vi "BDF-Read Record For Playback.vi"(0 "Header":T1, 5 "refnum in":refnum<file>, 9 "TCP samples":i32, 11 "error in (no error)":errorcluster) -> (6 "refnum out":refnum<file>, 8 "Array":u8[][](array[numeric]), 15 "error out":errorcluster)   [LabVIEW 2020]
uses:
  BDF-Header.ctl
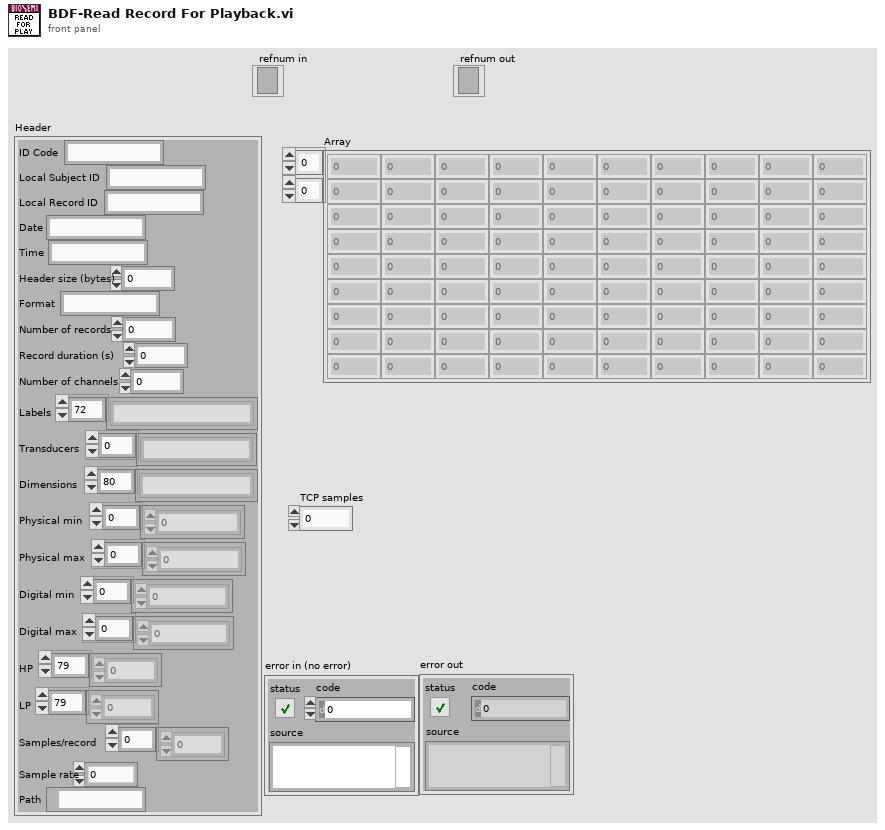
[diagram p1: front panel]
types:
  T1 = typedef "BDF-Header.ctl" = cluster{"ID Code":string, "Local Subject ID":string, "Local Record ID":string, "Date":string, "Time":string, "Header size (bytes)":i32, "Format":string, "Number of records":i32, "Record duration (s)":dbl, "Number of channels":i32, "Labels":string[], "Transducers":string[], "Dimensions":string[], "Physical min":dbl[], "Physical max":dbl[], "Digital min":i32[], "Digital max":i32[], "HP":dbl[], "LP":dbl[], "Samples/record":i32[], "Sample rate":dbl, "Path":path}
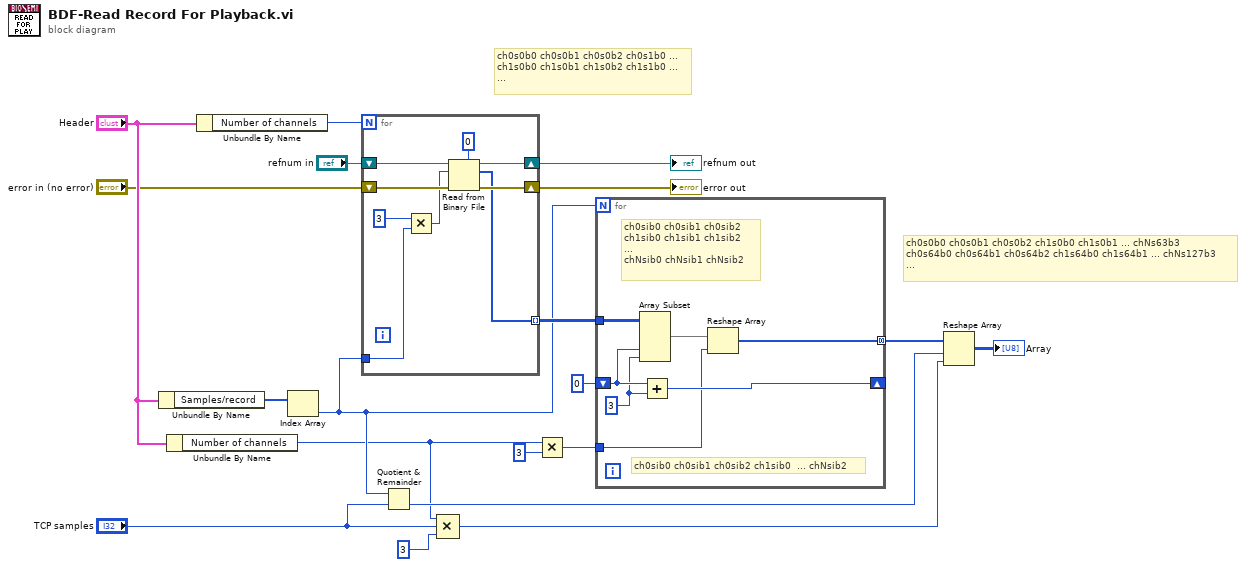
[diagram p0: block diagram]
diagram:
  # "ch0s0b0 ch0s0b1 ch0s0b2 ch1s0b0 ch1s0b1 ... chNs63b3\nch0s64b0 ch0s64b1 ch0s64b2 ch1s64b0 ch1s64b1 ... chNs127b3\n..."
  # "ch0s0b0 ch0s0b1 ch0s0b2 ch0s1b0 ...\nch1s0b0 ch1s0b1 ch1s0b2 ch1s1b0 ...\n..."
  n1 = Unbundle By Name("Header") -> ("Samples/record"=w17:i32[])
  n2 = Unbundle By Name("Header") -> ("Number of channels"=w5:i32)
  n3 = Unbundle By Name("Header") -> ("Number of channels"=w19:i32)
  n4 = Index Array(array=w17) -> (element=w6:i32)  [unwired: 1 in]
  n5 = for {
    N: w19 -> [_]
    tunnel: w6 -> [w20]
    shift-right: [w23] -> w3
    shift-left: "refnum in" -> [w28]
    shift-right: [w26] -> w1
    shift-left: "error in (no error)" -> [w27]
    tunnel: [w21] -> w8 mode=indexing
    n6 = Multiply(x=3, y=w20) -> (x*y=w24:i32)
    n7 = Read from Binary File(5:u8 0 ("Numeric"), 8:w27, 10:w24, 11:w28) -> (0:w26:errorcluster, 2:w21:u8[], 3:w23:refnum<file>)  [unwired: 2 in, 1 out]
  }
  "error out" <- w1
  "refnum out" <- w3
  n8 = Quotient & Remainder(x=w6, y="TCP samples") -> (floor(x/y)=w10:i32)  [unwired: 1 out]
  n9 = Compound Arithmetic op=MULTIPLY(w5, "TCP samples", 3 ("y")) -> (w12:i32)
  n10 = Multiply(x=w5, y=3) -> (x*y=w14:i32)
  n11 = for {
    N: w6 -> [_]
    tunnel: w8 -> [w35]
    shift-right: [w32] -> _
    shift-left: 0 -> [w34]
    tunnel: [w30] -> w7 mode=concatenating
    tunnel: w14 -> [w29]
    w33 = 3 ("length")
    # "ch0sib0 ch0sib1 ch0sib2 ch1sib0  ... chNsib2"
    # "ch0sib0 ch0sib1 ch0sib2\nch1sib0 ch1sib1 ch1sib2\n...\nchNsib0 chNsib1 chNsib2"
    n12 = Array Subset(array=w35, index (col)=w34, length (col)=w33) -> (w31:u8[][])  [unwired: 2 in]
    n13 = Add(x=w34, y=w33) -> (x+y=w32:i32)
    n14 = Reshape Array(w31, w29) -> (w30:u8[])
  }
  n15 = Reshape Array(w7, w10, w12) -> (→"Array":u8[][])
